vi "Wait For Command.vi"(8 "error in (no error)":errorcluster, 9 "timeout in ms (0)":i32 format="%d ms", 11 "Plugin Thread in":refnum<class "Plugin Thread.lvclass">) -> (0 "error out":errorcluster, 2 "command":T1={"Command"=enum."Start", "Parameters"={"arg1"=0, "arg2"=0}}, 3 "Plugin Thread out":refnum<class "Plugin Thread.lvclass">)   [LabVIEW 2017, in "DSF Core.lvlib" / "Plugin Thread.lvclass"]
uses:
  Plugin Thread.lvclass
  C:/Git/DSF/Core/Classes/Thread/Thread.lvclass
  Command Data.ctl
  Commands.ctl
  Interface/Plugin/Command Parameters.ctl
  Plugin Thread.lvclass/Plugin Thread.ctl
  Interface/Plugin/Response.ctl
  Interface/Plugin/Response Data.ctl
  Interface/Plugin/Response Parameters.ctl
  Thread.lvclass
  Interface/Plugin/Plugin Interface.lvclass
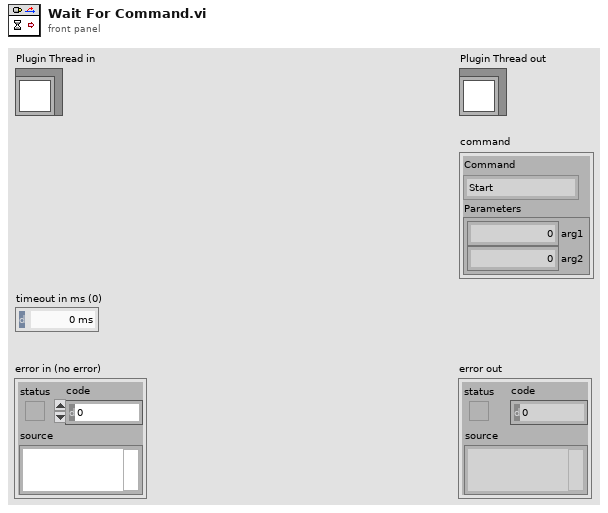
[diagram p1: front panel]
types:
  T1 = typedef "DSF Core.lvlib/Plugin Thread.lvclass/Command Data.ctl" = cluster{"Command":T2, "Parameters":T3}
  T2 = typedef "DSF Core.lvlib/Plugin Thread.lvclass/Commands.ctl" = enum8{"Idle", "Error", "Start", "Rx", "Tx", "Shutdown"}
  T3 = typedef "DSF Core.lvlib/Plugin Interface.lvclass/Command Parameters.ctl" = cluster{"arg1":u64, "arg2":u64}
  T4 = typedef "DSF Core.lvlib/Plugin Interface.lvclass/Command Data.ctl" = cluster{"Command":T5, "Parameters":T3}
  T5 = typedef "DSF Core.lvlib/Plugin Interface.lvclass/Command.ctl" = enum8{"Idle", "Start", "Set Inline Buffer", "Rx", "Tx", "Shutdown", "Error"}
  T6 = typedef "DSF Core.lvlib/Plugin Interface.lvclass/Response.ctl" = enum8{"General Ack", "Shutting Down"}
  T7 = typedef "DSF Core.lvlib/Plugin Interface.lvclass/Response Data.ctl" = cluster{"Response":T6, "Parameters":T8}
  T8 = typedef "DSF Core.lvlib/Plugin Interface.lvclass/Response Parameters.ctl" = cluster{"arg1":u64, "arg2":u64}
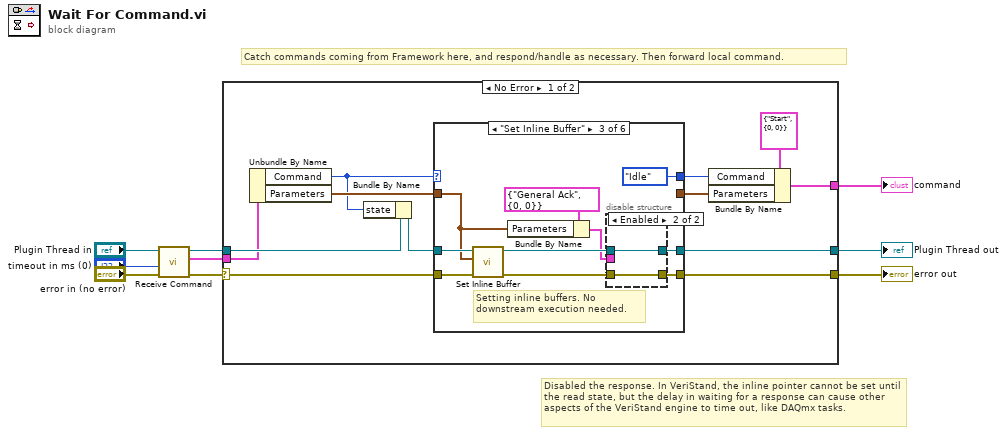
[diagram p0: block diagram]
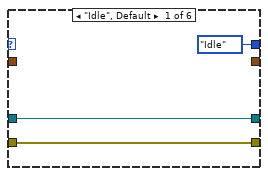
[diagram p2: hidden frame]
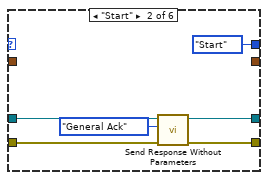
[diagram p3: hidden frame]
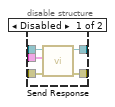
[diagram p4: hidden frame]
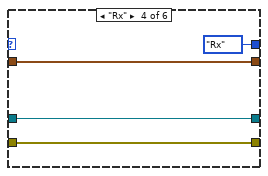
[diagram p5: hidden frame]
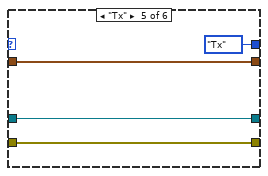
[diagram p6: hidden frame]
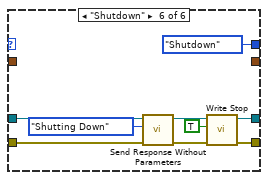
[diagram p7: hidden frame]
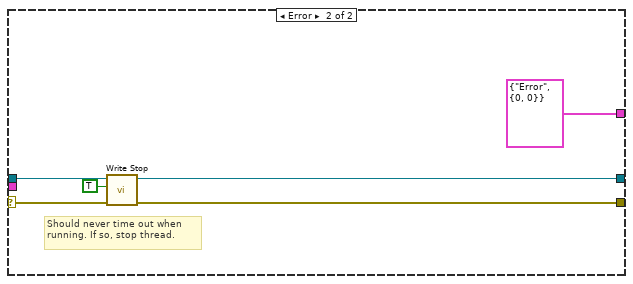
[diagram p8: hidden frame]
diagram:
  # "Disabled the response. In VeriStand, the inline pointer cannot be set until the read state, but the delay in waiting for a response can cause other aspects of the VeriStand engine to time out, like DAQmx tasks."
  # "Catch commands coming from Framework here, and respond/handle as necessary. Then forward local command."
  n1 = call "Receive Command.vi"("error in (no error)"="error in (no error)", "timeout in ms (0)"="timeout in ms (0)", "Plugin Thread in"="Plugin Thread in") -> ("error out"=w6:errorcluster, "command"=w2:T4, "Plugin Thread out"=w4:refnum<class "Plugin Thread.lvclass">)  [unwired: 6 in]
  n2 = case shown="No Error" w6 {
    selector: w6 -> [w20 w69]
    tunnel: [w18 w68] -> w5
    tunnel: w4 -> [w14 w67]
    tunnel: [w19 w66] -> w3
    tunnel: w2 -> [w11 _]
    tunnel: [w16 T1 {"Command"=enum."Error", "Parameters"={"arg1"=0, "arg2"=0}} ("Command")] -> w1
    frame No Error {
      n3 = Unbundle By Name(w11) -> ("Command"=w10:T5, "Parameters"=w13:T3)
      n4 = Bundle By Name(cluster=w14, "state"=w10) -> (w21:refnum<class "Plugin Thread.lvclass">)
      n5 = case shown="\"Set Inline Buffer\"" w10 {
        tunnel: w21 -> [w24 w29 w39 w50 w54 w61]
        tunnel: w20 -> [w23 w26 w38 w49 w53 w60]
        tunnel: [w24 w28 w34 w50 w54 w58] -> w19
        tunnel: [w23 w27 w35 w49 w53 w56] -> w18
        tunnel: [Commands."Idle" ("command") Commands."Start" ("command") Commands."Idle" ("command") Commands."Rx" ("command") Commands."Tx" ("command") Commands."Shutdown" ("command")] -> w15
        tunnel: w13 -> [_ _ w31 w51 w55 _]
        tunnel: [_ _ _ w51 w55 _] -> w12
        frame "Idle", Default {
        }
        frame "Start" {
          n6 = call "Send Response Without Parameters.vi"("error in (no error)"=w26, "response"=Response."General Ack", "Plugin Thread in"=w29) -> ("error out"=w27:errorcluster, "Plugin Thread out"=w28:refnum<class "Plugin Thread.lvclass">)  [unwired: 7 in]
        }
        frame "Set Inline Buffer" {
          # "Setting inline buffers. No downstream execution needed."
          n7 = call "Set Inline Buffer.vi"("error in (no error)"=w38, "command parameters"=w31, "Plugin Thread in"=w39) -> ("error out"=w37:errorcluster, "Plugin Thread out"=w36:refnum<class "Plugin Thread.lvclass">)  [unwired: 7 in]
          n8 = Bundle By Name(cluster=T7 {"Response"=enum."General Ack", "Parameters"={"arg1"=0, "arg2"=0}} ("response"), "Parameters"=w31) -> (w32:T7)
          n9 = disable-structure shown="Enabled" {
            disable-tunnel: w37 -> [w45 w47]
            disable-tunnel: w36 -> [w44 w46]
            disable-tunnel: [w43 w47] -> w35
            disable-tunnel: [w42 w46] -> w34
            disable-tunnel: w32 -> [w41 _]
            frame Disabled {
              n10 = call "Send Response.vi"("error in (no error)"=w45, "response"=w41, "Plugin Thread in"=w44) -> ("error out"=w43:errorcluster, "Plugin Thread out"=w42:refnum<class "Plugin Thread.lvclass">)  [unwired: 7 in]
            }
            frame Enabled {
            }
          }
        }
        frame "Rx" {
        }
        frame "Tx" {
        }
        frame "Shutdown" {
          n11 = call "Send Response Without Parameters.vi"("error in (no error)"=w60, "response"=Response."Shutting Down", "Plugin Thread in"=w61) -> ("error out"=w57:errorcluster, "Plugin Thread out"=w59:refnum<class "Plugin Thread.lvclass">)  [unwired: 7 in]
          n12 = call "Write Stop.vi"("error in (no error)"=w57, "stop"=TRUE, "Thread in"=w59) -> ("error out"=w56:errorcluster, "Thread out"=w58:refnum<class "Plugin Thread.lvclass">)  [unwired: 7 in]
        }
      }
      n13 = Bundle By Name(cluster=T1 {"Command"=enum."Start", "Parameters"={"arg1"=0, "arg2"=0}} ("Command"), "Command"=w15, "Parameters"=w12) -> (w16:T1)
    }
    frame Error {
      # "Should never time out when running. If so, stop thread."
      n14 = call "Write Stop.vi"("error in (no error)"=w69, "stop"=TRUE, "Thread in"=w67) -> ("error out"=w68:errorcluster, "Thread out"=w66:refnum<class "Plugin Thread.lvclass">)  [unwired: 7 in]
    }
  }
  "error out" <- w5
  "Plugin Thread out" <- w3
  "command" <- w1
